vi "Load Classes.vi"(8 "error in (no error)":errorcluster, 10 "class paths":path[](array[path]), 11 "Class Loader in":refnum<class "Class Loader.lvclass">) -> (0 "error out":errorcluster, 2 "objects":refnum<class>[](array[class]), 3 "Class Loader out":refnum<class "Class Loader.lvclass">)   [LabVIEW 2017, in "Data Sharing Framework Engine.lvlib" / "Class Loader.lvclass"]
uses:
  Class Loader.lvclass
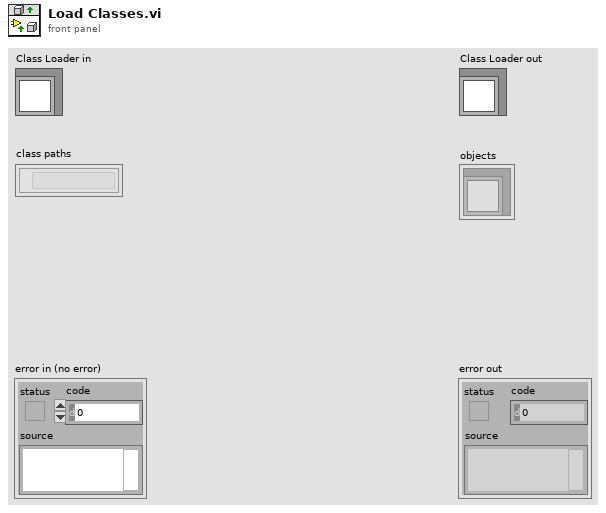
[diagram p1: front panel]
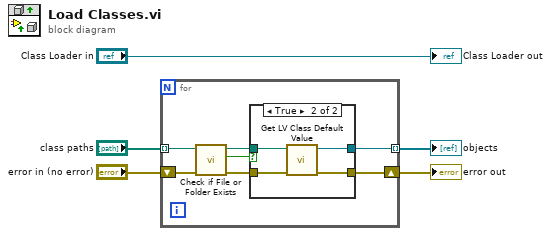
[diagram p0: block diagram]
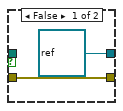
[diagram p2: hidden frame]
diagram:
  n1 = for {
    shift-right: [w7] -> w3
    shift-left: "error in (no error)" -> [w12]
    tunnel: "class paths" -> [w11] mode=indexing
    tunnel: [w6] -> w2 mode=indexing
    n2 = call <vilib>:"Check if File or Folder Exists.vi"("error in (no error)"=w12, "path"=w11) -> ("error out"=w9:errorcluster, "file or folder exists?"=w10:bool, "dup path"=w8:path)  [unwired: 7 in]
    n3 = case shown="True" w10 {
      tunnel: w9 -> [w13 w18]
      tunnel: w8 -> [_ w17]
      tunnel: [refnum<class> refnum ("object") w16] -> w6
      tunnel: [w13 w15] -> w7
      frame False {
      }
      frame True {
        n4 = call <vilib>:"Get LV Class Default Value.vi"("error in (no error)"=w18, "class path"=w17) -> ("error out"=w15:errorcluster, "object"=w16:refnum<class>)  [unwired: 8 in]
      }
    }
  }
  "error out" <- w3
  "objects" <- w2
  "Class Loader out" <- "Class Loader in"
